vi "SelectFile.vi"(8 "Error In":errorcluster, 9 "File Description":string="All Files", 10 "File Extension (.*)":string=".*", 11 "Start Path":path) -> (0 "Error Out":errorcluster, 2 "Cancelled?":bool caption="cancelled", 3 "Selected File Path":path)   [LabVIEW 2012, in "Virtual-PGA.lvlib"]
uses:
  Virtual-PGA.lvlib
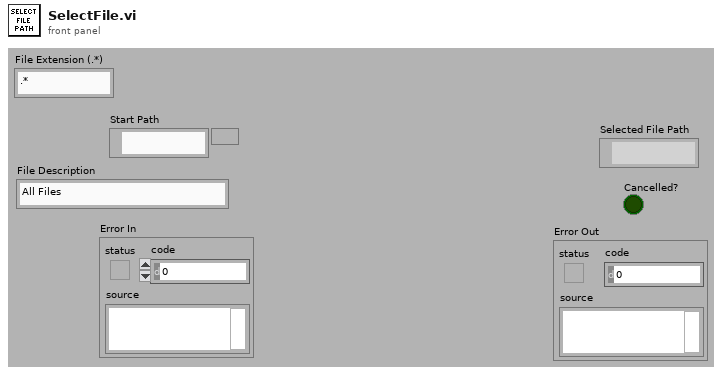
[diagram p1: front panel]
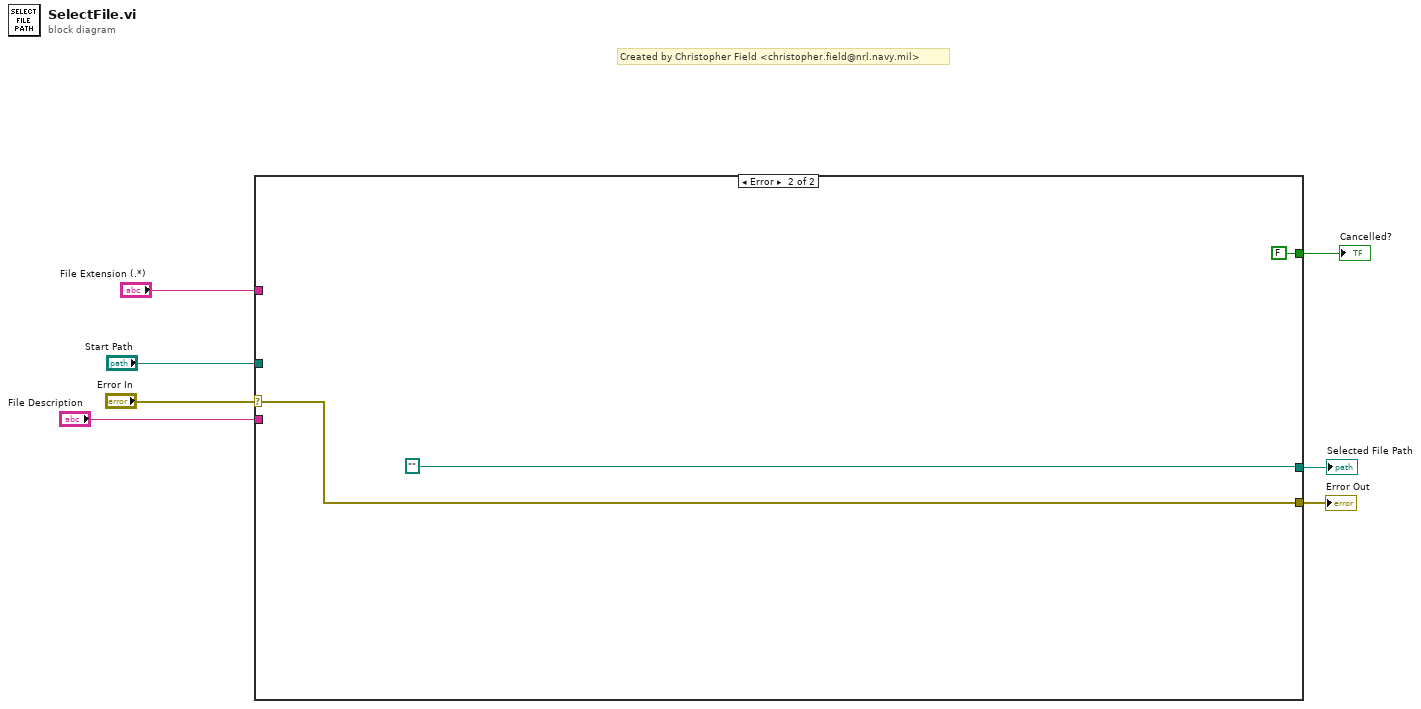
[diagram p0: block diagram]
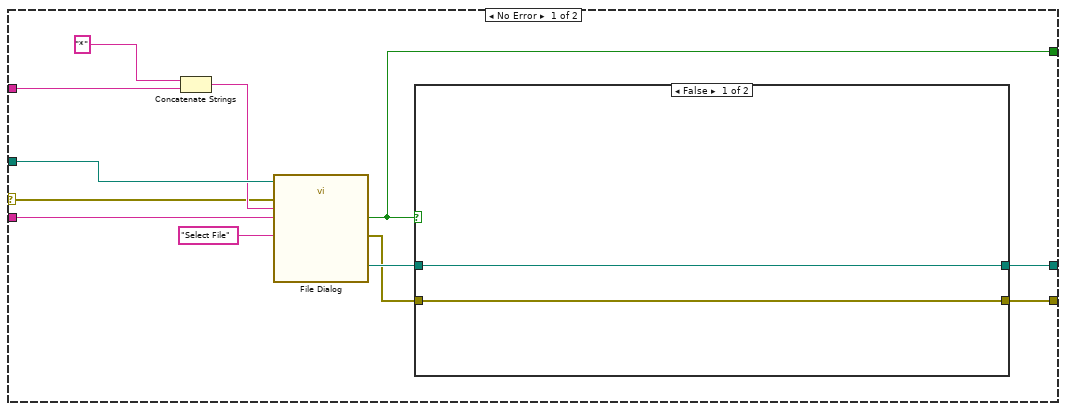
[diagram p2: hidden frame]
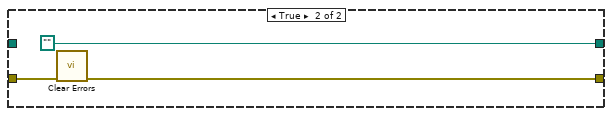
[diagram p3: hidden frame]
diagram:
  # "Created by Christopher Field <christopher.field@nrl.navy.mil>"
  n1 = case shown="Error" "Error In" {
    selector: "Error In" -> [w8 w26]
    tunnel: "Start Path" -> [w19 _]
    tunnel: "File Description" -> [w18 _]
    tunnel: [w16 FALSE ("cancelled")] -> w5
    tunnel: [w13 w26] -> w4
    tunnel: [w12 path ""] -> w3
    tunnel: "File Extension (.*)" -> [w10 _]
    frame No Error {
      n2 = Concatenate Strings("*" ("string"), w10) -> (w9:string)
      n3 = call "File Dialog"("start path"=w19, "prompt"="Select File", "error in"=w8, "pattern (all files)"=w9, "pattern label"=w18) -> ("selected path"=w15:path, "cancelled"=w16:bool, "error out"=w14:errorcluster)  [unwired: 7 in, 1 out]
      n4 = case shown="False" w16 {
        tunnel: w15 -> [w20 _]
        tunnel: w14 -> [w21 w24]
        tunnel: [w21 w23] -> w13
        tunnel: [w20 path ""] -> w12
        frame False {
        }
        frame True {
          n5 = call <vilib>:"Clear Errors.vi"("error in (no error)"=w24) -> ("error out"=w23:errorcluster)  [unwired: 6 in]
        }
      }
    }
    frame Error {
    }
  }
  "Cancelled?" <- w5
  "Error Out" <- w4
  "Selected File Path" <- w3
